vi "load new file.vi"(6 "Path":path, 7 "View":T3, 8 "error in (no error)":errorcluster, 11 "Application Refs":T1) -> (0 "error out":errorcluster, 3 "Application Data out":T1)   [LabVIEW 2017]
uses:
  View Mode.ctl
  Application Data.ctl
  DSF Configuration API/1.0.0/Public/Controls/DSF Config Data RefNum.ctl
  Window State.ctl
  DSF Configuration API/1.0.0/DSF Configuration API.lvlib
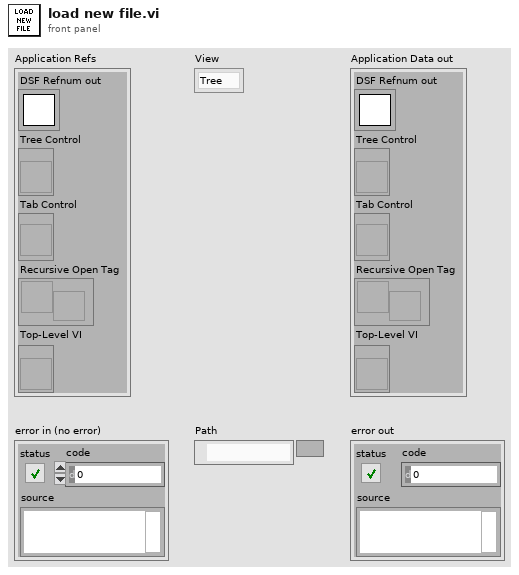
[diagram p1: front panel]
types:
  T1 = typedef "Application Data.ctl" = cluster{"DSF Refnum out":T2, "Tree Control":refnum<vi>, "Tab Control":refnum<vi>, "Recursive Open Tag":refnum<user-event>, "Top-Level VI":refnum<vi>}
  T2 = typedef "DSF Configuration API.lvlib/DSF Config Data RefNum.ctl" = refnum<k1>
  T3 = typedef "View Mode.ctl" = enum16{"Tree", "List"}
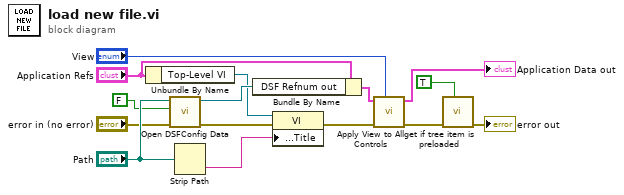
[diagram p0: block diagram]
diagram:
  n1 = Unbundle By Name("Application Refs") -> ("Top-Level VI"=w4:refnum<vi>)
  n2 = call "Open DSFConfig Data.vi"("error in (no error)"="error in (no error)", "create file if necessary (T)"=FALSE, "configuration file path"="Path") -> ("error out"=w14:errorcluster, "refnum"=w8:T2)  [unwired: 5 in, 2 out]
  n3 = Strip Path(path="Path") -> (name=w13:string)  [unwired: 1 out]
  n4 = Bundle By Name(cluster="Application Refs", "DSF Refnum out"=w8) -> (w7:T1)
  n5 = property class="VI"(reference=w4, error in=w14, "Front Panel.Title"=w13) -> (error out=w15:errorcluster)  [unwired: 1 out]
  n6 = call "Apply View to All Controls.vi"("View Mode"="View", "error in (no error)"=w15, "Application Data in"=w7) -> ("error out"=w3:errorcluster, "Application Data out"=→"Application Data out":T1)  [unwired: 7 in]
  n7 = call "get if tree item is preloaded.vi"("clear entries"=TRUE, "error in (no error)"=w3) -> ("error out"=→"error out":errorcluster)  [unwired: 7 in, 2 out]
